vi "Shorten common factors.vi"(10 "Denumerator in":i64, 11 "Numerator in":i64) -> (2 "Denumerator out":i64, 3 "Numerator out":i64)   [LabVIEW 2021, in "Rational Number.lvclass"]
uses:
  Rational Number.lvclass
  <vilib>/gmath/NI_Gmath.lvlib
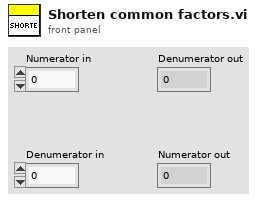
[diagram p1: front panel]
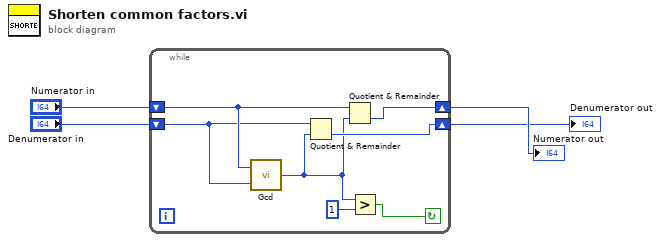
[diagram p0: block diagram]
diagram:
  n1 = while {
    shift-right: [w10] -> w4
    shift-left: "Numerator in" -> [w11]
    shift-right: [w8] -> w3
    shift-left: "Denumerator in" -> [w9]
    stop <- w5 continue-if-true
    n2 = call <vilib>:"Gcd.vi"("y"=w9, "x"=w11) -> ("gcd(x,y)"=w7:i32)
    n3 = Quotient & Remainder(x=w9, y=w7) -> (floor(x/y)=w8:i64)  [unwired: 1 out]
    n4 = Quotient & Remainder(x=w11, y=w7) -> (floor(x/y)=w10:i64)  [unwired: 1 out]
    n5 = Greater?(x=w7, y=1) -> (0:w5:bool)
  }
  "Numerator out" <- w4
  "Denumerator out" <- w3
